vi "chartsheet set chart opt.vi"(8 "error in (no error)":errorcluster, 9 "options":T1, 10 "chart":u32, 11 "chartsheet":u32) -> (0 "error out":errorcluster, 1 "options out":T1, 3 "function return":u32(ring))   [LabVIEW 2015, in "xlsxwriter.lvlib"]
doc: "lxw_error chartsheet_set_chart_opt(lxw_chartsheet chartsheet, lxw_chart chart, lxw_chart_options *options);"
uses:
  xlsxwriter.lvlib
  xlsxwriter.dll
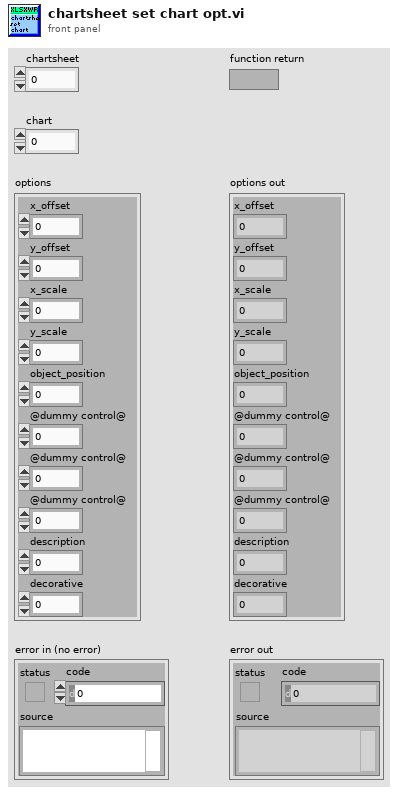
[diagram p1: front panel]
types:
  T1 = cluster{"x_offset":i32, "y_offset":i32, "x_scale":dbl, "y_scale":dbl, "object_position":u8, "@dummy control@":i8, "@dummy control@":i8, "@dummy control@":i8, "description":u32, "decorative":u32}
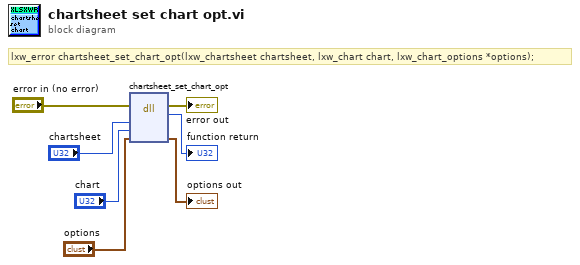
[diagram p0: block diagram]
diagram:
  # "lxw_error chartsheet_set_chart_opt(lxw_chartsheet chartsheet, lxw_chart chart, lxw_chart_options *options);"
  n1 = dll-call lib="C:/Users/WDAGUtilityAccount/Desktop/lv_vis_added_cell/xlsxwriter.*" fn="chartsheet_set_chart_opt"(error in="error in (no error)", "chartsheet"="chartsheet", "chart"="chart", "options"="options") -> (error out=→"error out":errorcluster, →"function return":u32, "options"=→"options out":T1)  [unwired: 4 in, 1 out]
